vi "ControlFileToVariant.vi"(8 "error in":errorcluster, 11 "State":T1) -> (0 "error out":errorcluster, 3 "State out":T1)   [LabVIEW 2013, in "data interface script.lvlib"]
uses:
  data interface script.lvlib
  Controls/StateCluster.ctl
  Controls/initialized references.ctl
  Controls/interface VI type.ctl
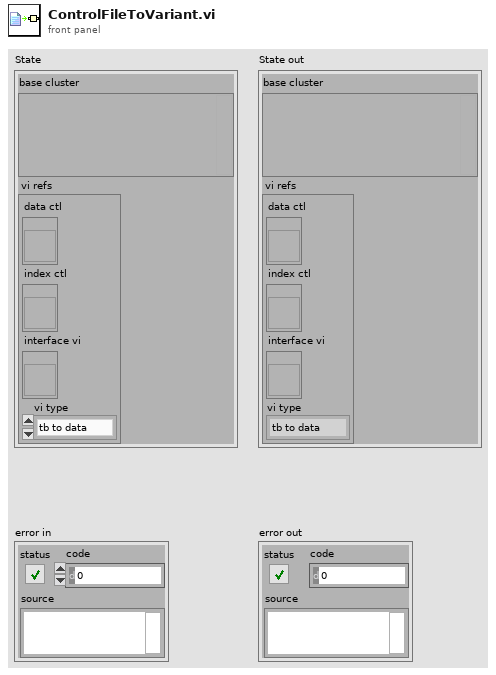
[diagram p1: front panel]
types:
  T1 = typedef "data interface script.lvlib/StateCluster.ctl" = cluster{"base cluster":variant, "vi refs":T2}
  T2 = typedef "data interface script.lvlib/initialized references.ctl" = cluster{"data ctl":refnum<vi>, "index ctl":refnum<vi>, "interface vi":refnum<vi>, "vi type":T3}
  T3 = typedef "data interface script.lvlib/interface VI type.ctl" = enum16{"tb to data", "data to tb"}
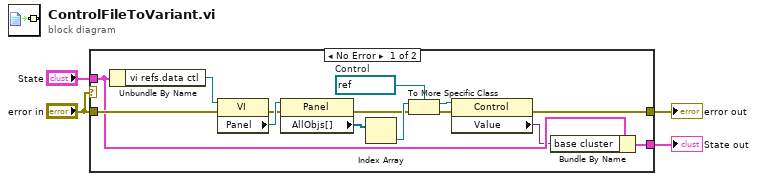
[diagram p0: block diagram]
diagram:
  n1 = case shown="No Error" "error in" {
    tunnel: [w18 w20] -> w4
    tunnel: "error in" -> [w17 w20]
    tunnel: "State" -> [w9 w19]
    tunnel: [w7 w19] -> w2
    frame No Error {
      w16 = refnum<vi> refnum  # Control
      n2 = Unbundle By Name(w9) -> ("vi refs.data ctl"=w5:refnum<vi>)
      n3 = property class="VI"(reference=w5, error in=w17) -> (error out=w10:errorcluster, "Panel"=w11:refnum<vi>)  [unwired: 1 out]
      n4 = property class="Panel"(reference=w11, error in=w10) -> (error out=w6:errorcluster, "AllObjs[]"=w12:refnum<vi>[])  [unwired: 1 out]
      n5 = Index Array(array=w12) -> (element=w14:refnum<vi>)  [unwired: 1 in]
      n6 = To More Specific Class(target class=w16, reference=w14, error in=w6) -> (specific class reference=w15:refnum<vi>, error out=w13:errorcluster)
      n7 = property class="Control"(reference=w15, error in=w13) -> (error out=w18:errorcluster, "Value"=w8:variant)  [unwired: 1 out]
      n8 = Bundle By Name(cluster=w9, "base cluster"=w8) -> (w7:T1)
    }
    frame Error {
    }
  }
  "error out" <- w4
  "State out" <- w2
